vi "NI VeriStand - Set Alarm Mode.vi"(8 "error in (no error)":errorcluster, 10 "Alarm Mode":u8(ring) items=["Normal", "Indicate Only"], 11 "Alarm in":T1) -> (0 "error out":errorcluster, 3 "Alarm out":T1)   [LabVIEW 2020, in "NI_VS Alarm ExecutionAPI.lvlib"]
doc: "Sets the operating mode of the specified alarm."
uses:
  <vilib>/NI VeriStand/Execution/Alarm/NI_VS Alarm ExecutionAPI.lvlib
  <vilib>/NI VeriStand/Execution/Alarm/AlarmAPI.ctl
  NationalInstruments.VeriStand.ClientAPI
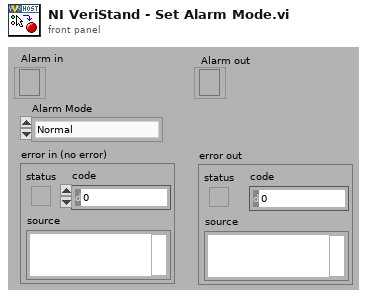
[diagram p1: front panel]
types:
  T1 = typedef "NI_VS Alarm ExecutionAPI.lvlib/AlarmAPI.ctl" = refnum<k24>
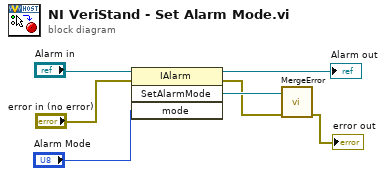
[diagram p0: block diagram]
diagram:
  n1 = invoke class="IAlarm" method="SetAlarmMode"(reference="Alarm in", error in="error in (no error)", "mode"="Alarm Mode") -> (reference out=→"Alarm out":T1, error out=w3:errorcluster, "SetAlarmMode"=w5:refnum<k24>)  [unwired: 1 in, 1 out]
  n2 = call <vilib>:"MergeError.vi"("error in (no error)"=w3, "Error"=w5) -> ("error out"=→"error out":errorcluster)  [unwired: 9 out]
